vi "niScope Property Node.vi"   [LabVIEW 2013]
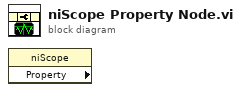
[diagram p0: block diagram]
diagram:
  n1 = property class="niScope" props=[]() -> ()  [unwired: 2 in, 3 out]
